vi "Close.vi"(8 "error in":errorcluster, 11 "MeasureLimit":refnum<class "MeasureLimit.lvclass">) -> (0 "error out":errorcluster)   [LabVIEW 2021, in "ProligentXMLGenerator.lvlib" / "MeasureLimit.lvclass"]
uses:
  MeasureLimit.lvclass
  MeasureLimit.lvclass/MeasureLimit.ctl
  Model/CustomData/CustomData.lvclass
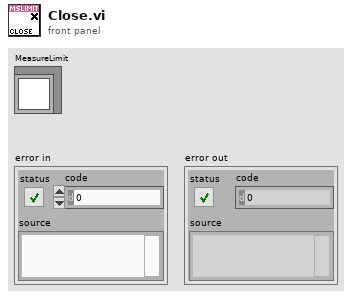
[diagram p1: front panel]
types:
  T1 = typedef "ProligentXMLGenerator.lvlib/MeasureLimit.lvclass/Data.ctl" = cluster{"Name":string, "CustomData":refnum<class "CustomData.lvclass">, "LimitExpression":refnum<class "NonEmptyString_2000.lvclass">}
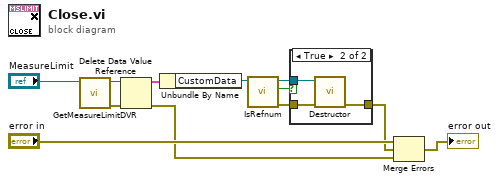
[diagram p0: block diagram]
diagram:
  n1 = call "GetMeasureLimitDVR.vi"("MeasureLimit"="MeasureLimit") -> ("error out"=w9:errorcluster, "DVRReference"=w10:refnum<data-value>)  [unwired: 9 in]
  n2 = Delete Data Value Reference(data value reference=w10, error in=w9) -> (data value=w3:T1, error out=w8:errorcluster)
  n3 = Unbundle By Name(w3) -> ("CustomData"=w2:refnum<class "CustomData.lvclass">)
  n4 = call "IsRefnum.vi"("CustomDataType in"=w2) -> ("error out"=w6:errorcluster, "IsRefnum"=w5:bool, "CustomDataType out"=w4:refnum<class "CustomData.lvclass">)  [unwired: 8 in]
  n5 = case shown="True" w5 {
    tunnel: w6 -> [w13 w16]
    tunnel: [w13 w15] -> w1
    tunnel: w4 -> [_ w14]
    frame False {
    }
    frame True {
      n6 = call "Destructor.vi"("error in"=w16, "CustomDataType"=w14) -> ("error out"=w15:errorcluster)  [unwired: 9 in]
    }
  }
  n7 = Merge Errors("error in", w1, w8) -> (→"error out":errorcluster)
